vi "Load Controller Type from Path.vi"(2 "error in (no error)":errorcluster, 3 "Class Path":path) -> (0 "error out":errorcluster, 1 "Controller out":refnum<class "Generic Plugin.lvclass">)   [LabVIEW 2020, in "RxnRover.lvlib" / "Generic Plugin.lvclass"]
doc: "Loads the plugin server class from the provided path. This should be an absolute path in the development environment and a relative path for standalone applications."
uses:
  Generic Plugin.lvclass
  Pump Controller/Pump Controller.lvclass
  logging/logging.lvlib
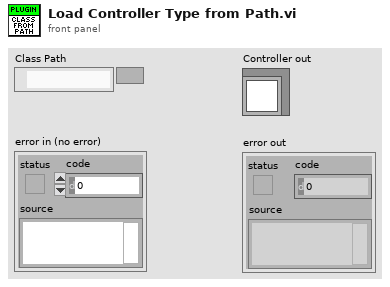
[diagram p1: front panel]
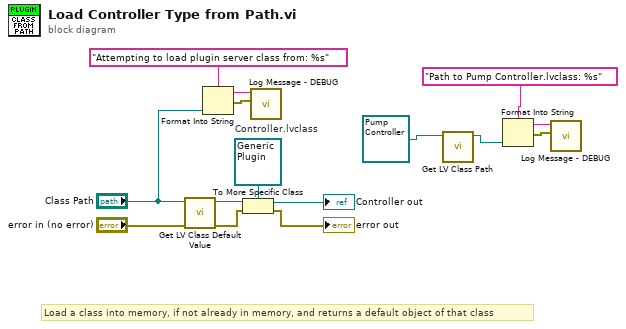
[diagram p0: block diagram]
diagram:
  w13 = refnum<class "Generic Plugin.lvclass"> refnum  # Controller.lvclass
  # "Load a class into memory, if not already in memory, and returns a default object of that class"
  n1 = call <vilib>:"Get LV Class Default Value.vi"("error in (no error)"="error in (no error)", "class path"="Class Path") -> ("error out"=w7:errorcluster, "object"=w14:refnum<class>)  [unwired: 8 in]
  n2 = Format Into String(format string="Attempting to load plugin server class from: %s", "Class Path") -> (resulting string=w9:string, error out=w10:errorcluster)  [unwired: 2 in]
  n3 = To More Specific Class(target class=w13, reference=w14, error in=w7) -> (specific class reference=→"Controller out":refnum<class "Generic Plugin.lvclass">, error out=→"error out":errorcluster)
  n4 = call "Log Message - DEBUG.vi"("error in (no error)"=w10, "Message"=w9) -> ()  [unwired: 9 in, 1 out]
  n5 = call <vilib>:"Get LV Class Path.vi"("object"=refnum<class "Pump Controller.lvclass"> refnum ("RxnRover.lvlib:Pump Controller.lvclass")) -> ("class path"=w2:path)  [unwired: 9 in, 1 out]
  n6 = Format Into String(format string="Path to Pump Controller.lvclass: %s", w2) -> (resulting string=w3:string, error out=w4:errorcluster)  [unwired: 2 in]
  n7 = call "Log Message - DEBUG.vi"("error in (no error)"=w4, "Message"=w3) -> ()  [unwired: 9 in, 1 out]
